vi "Wire Class to Enqueue.vi"(7 "Class Type":enum16{"Concrete", "Abstract"}(ring), 8 "error in (no error)":errorcluster, 10 "Message Object":refnum<vi>, 11 "vi reference":refnum<vi>) -> (0 "error out":errorcluster, 3 "dup VI Refnum":refnum<vi>)   [LabVIEW 2020, in "Message Maker.lvlib"]
uses:
  Message Maker.lvlib
  <vilib>/Utility/traverseref.llb/TRef TravTarget.ctl
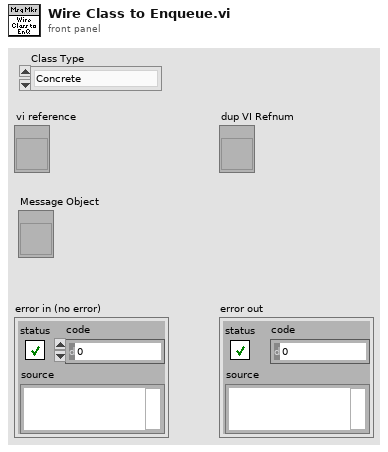
[diagram p1: front panel]
types:
  T1 = typedef "TRef TravTarget.ctl" = enum16{"FP", "BD", "Other"}
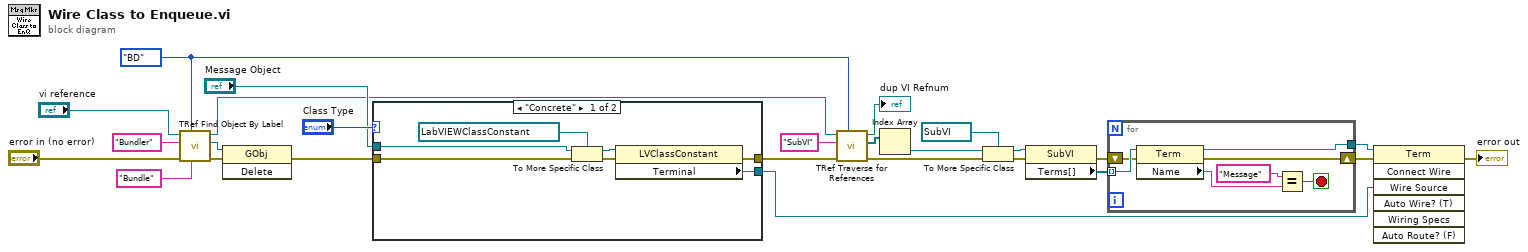
[diagram p0: block diagram]
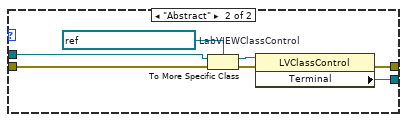
[diagram p2: hidden frame]
diagram:
  w9 = TRef_TravTarget."BD" ("Traverse Target")
  n1 = call <vilib>:"TRef Find Object By Label.vi"("Label"="Bundle", "Traverse Target"=w9, "error in (no error)"="error in (no error)", "Class Name"="Bundler", "VI Ref"="vi reference") -> ("error out"=w5:errorcluster, "Found Obj Ref"=w4:refnum<vi>, "dup VI Ref"=w2:refnum<vi>)  [unwired: 3 in, 1 out]
  n2 = invoke class="GObj" method="Delete"(reference=w4, error in=w5) -> (error out=w25:errorcluster)  [unwired: 1 in, 2 out]
  n3 = case shown="\"Concrete\"" "Class Type" {
    tunnel: w25 -> [w33 w40]
    tunnel: [w32 w35] -> w1
    tunnel: [w31 w34] -> w14
    tunnel: "Message Object" -> [w27 w39]
    frame "Concrete" {
      n4 = To More Specific Class(target class=refnum<vi> refnum ("element"), reference=w27, error in=w33) -> (specific class reference=w30:refnum<vi>, error out=w29:errorcluster)
      n5 = property class="LVClassConstant"(reference=w30, error in=w29) -> (error out=w32:errorcluster, "Terminal"=w31:refnum<vi>)  [unwired: 1 out]
    }
    frame "Abstract" {
      w38 = refnum<vi> refnum  # LabVIEWClassControl
      n6 = To More Specific Class(target class=w38, reference=w39, error in=w40) -> (specific class reference=w37:refnum<vi>, error out=w36:errorcluster)
      n7 = property class="LVClassControl"(reference=w37, error in=w36) -> (error out=w35:errorcluster, "Terminal"=w34:refnum<vi>)  [unwired: 1 out]
    }
  }
  n8 = call <vilib>:"TRef Traverse for References.vi"("Traverse Target"=w9, "error in (no error)"=w1, "Class Name"="SubVI", "VI Refnum"=w2) -> ("error out"=w16:errorcluster, "References"=w15:refnum<vi>[], "dup VI Refnum"=→"dup VI Refnum":refnum<vi>)  [unwired: 4 in, 1 out]
  n9 = Index Array(array=w15) -> (element=w23:refnum<vi>)  [unwired: 1 in]
  n10 = To More Specific Class(target class=refnum<vi> refnum ("element"), reference=w23, error in=w16) -> (specific class reference=w19:refnum<vi>, error out=w17:errorcluster)
  n11 = property class="SubVI"(reference=w19, error in=w17) -> (error out=w20:errorcluster, "Terms[]"=w21:refnum<vi>[])  [unwired: 1 out]
  n12 = for {
    tunnel: w21 -> [w47] mode=indexing
    shift-right: [w45] -> w18
    shift-left: w20 -> [w46]
    tunnel: [w44] -> w12
    stop <- w41 stop-if-true
    n13 = property class="Term"(reference=w47, error in=w46) -> (reference out=w44:refnum<vi>, error out=w45:errorcluster, "Name"=w42:string)
    n14 = Equal?(x="Message" ("element"), y=w42) -> (x = y?=w41:bool)
  }
  n15 = invoke class="Term" method="Connect Wire"(reference=w12, error in=w18, "Wire Source"=w14) -> (error out=→"error out":errorcluster)  [unwired: 4 in, 6 out]
